vi "lights work.vi"() -> ()   [LabVIEW 2016]
doc: "ADXL362 SPI Accelerometer\n\nThis example shows how to use the Analog Devices ADXL362 Accelerometer sensor connected to SPI.\n\nThis example expects a USB cable connected from your development PC to the Type B USB Jack (next to the power input) on the roboRIO."
uses:
  <vilib>/Rock Robotics/SystemInterfaces/spilib/spi_bus.ctl
  <vilib>/Rock Robotics/WPI/SPI/WPI_SPIMode.ctl
panel:
  out "Previous":i32[](array[numeric])
  out "ONOFF":bool
  in  "Blink Rate":u32
  in  "Aiming":u32(colorbox)
  in  "Loader":bool
  in  "Intake":bool
  in  "Shooter":bool
  in  "Blinky End":u8
  in  "Chaser (Gap)":u8
  in  "Display Style":u8(knob) scale=0.0..6.0
  out "Aiming":bool
  out "Loader":bool
  out "Intake":bool
  out "Shooter":bool
  in  "Global Max\nBrightness":u8(slide) max=31 scale=0.0..31.0
  in  "Brightness B":u8
  in  "Brighness R":u8
  in  "Brigtness G":u8
  in  "Blue":bool
  in  "Red":bool
  in  "Green":bool
  in  "Number of Lights":u8
  in  "Number ON":u8
  in  "Chip Select Active High (F)":bool
  in  "Mode (3)":T1=enum."Mode 3 (Clk Idle High,Sample on Trailing)"
  in  "Clock Rate (Hz)":dbl=500000.0
  in  "error in":errorcluster
  in  "SPI Bus":T2=enum."SPI On-Board, CS1"
  out "error out":errorcluster
  in  "stop":bool
  # "Set these inputs before running."
  # "Number of Lights"
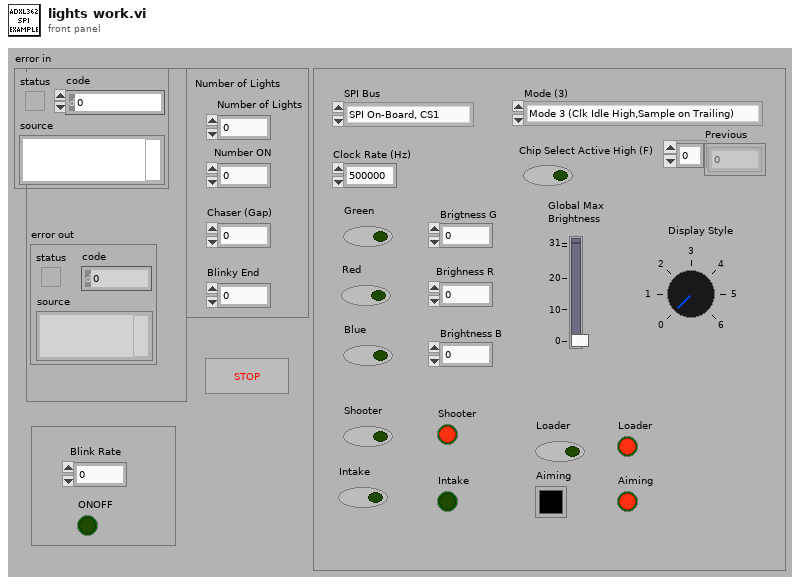
[diagram p1: front panel]
types:
  T1 = typedef "WPI_SPIMode.ctl" = enum16{"Mode 0 (Clk Idle Low,Sample on Leading)", "Mode 1 (Clk Idle Low,Sample on Trailing)", "Mode 2 (Clk Idle High,Sample on Leading)", "Mode 3 (Clk Idle High,Sample on Trailing)"}
  T2 = typedef "spi_bus.ctl" = enum16{"SPI On-Board, CS0", "SPI On-Board, CS1", "SPI On-Board, CS2", "SPI On-Board, CS3", "SPI MXP", "Invalid"}
  T3 = typedef "WPI_SPIDevRef.ctl" = cluster{"DevStatus":errorcluster, "Handle":i32, "SPI Bus":T2}
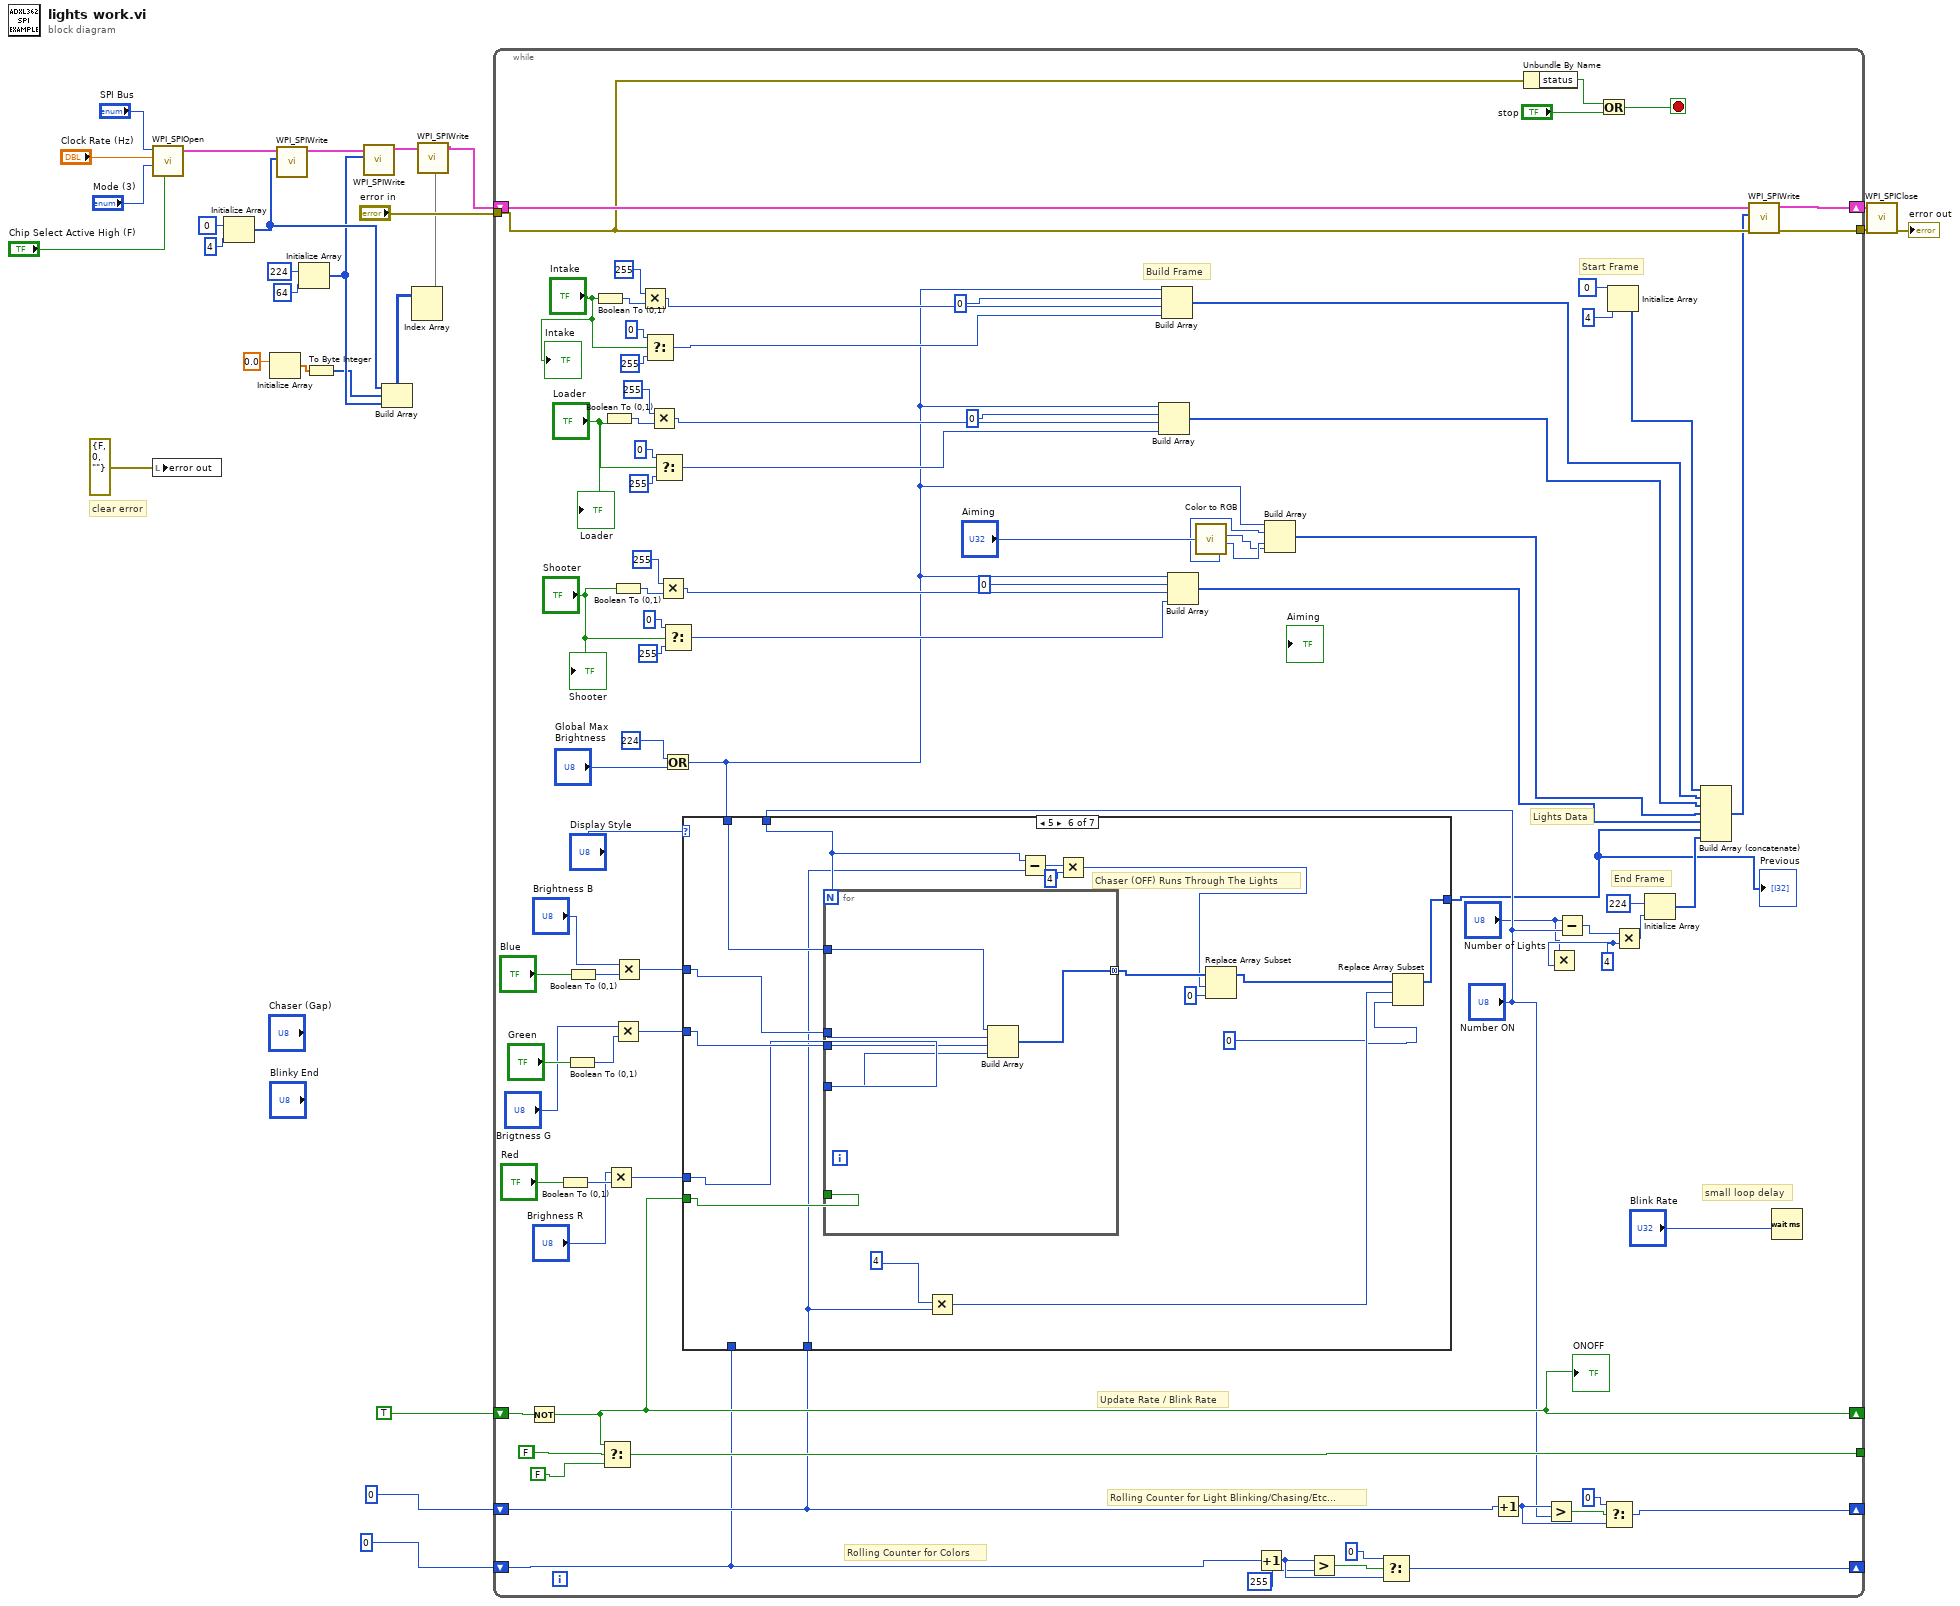
[diagram p0: block diagram]
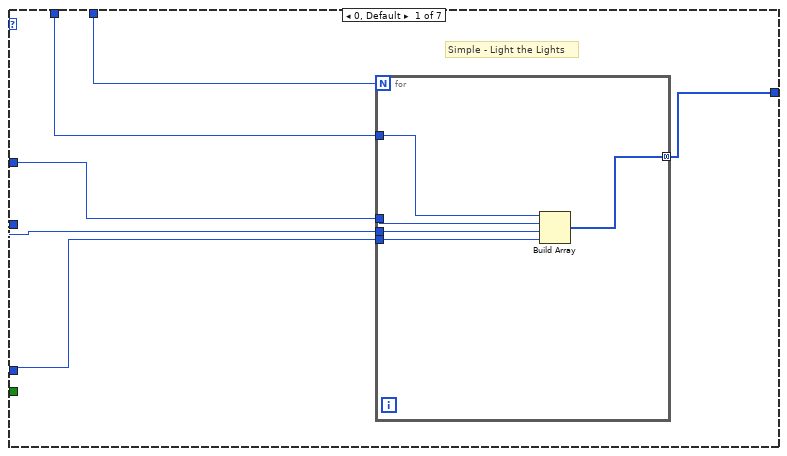
[diagram p2: hidden frame]
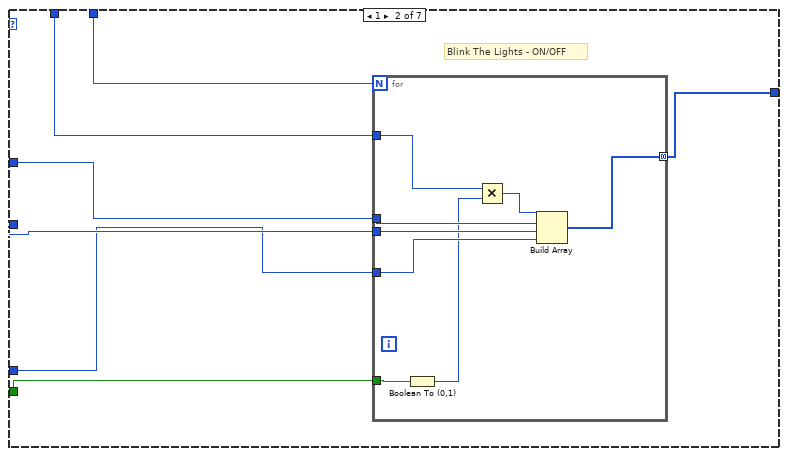
[diagram p3: hidden frame]
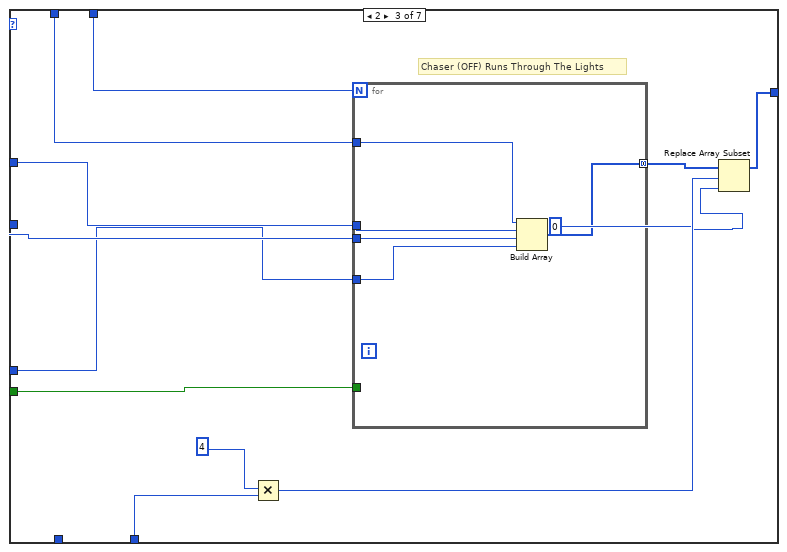
[diagram p4: hidden frame]
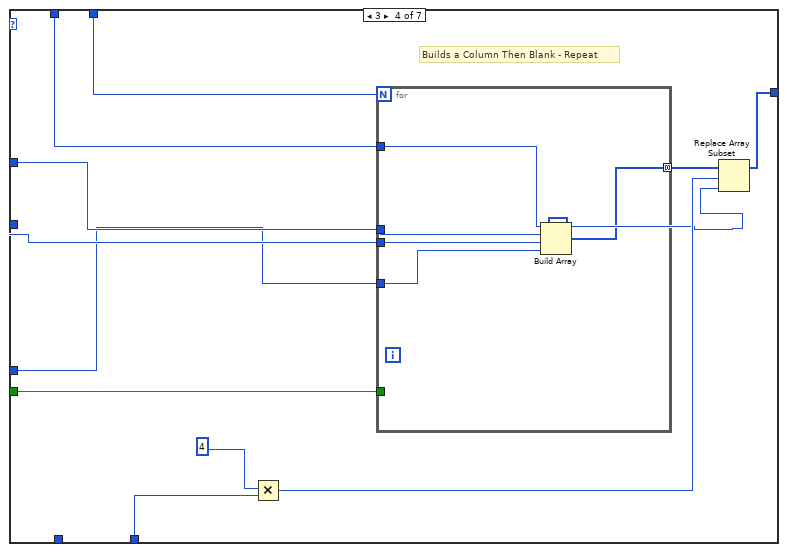
[diagram p5: hidden frame]
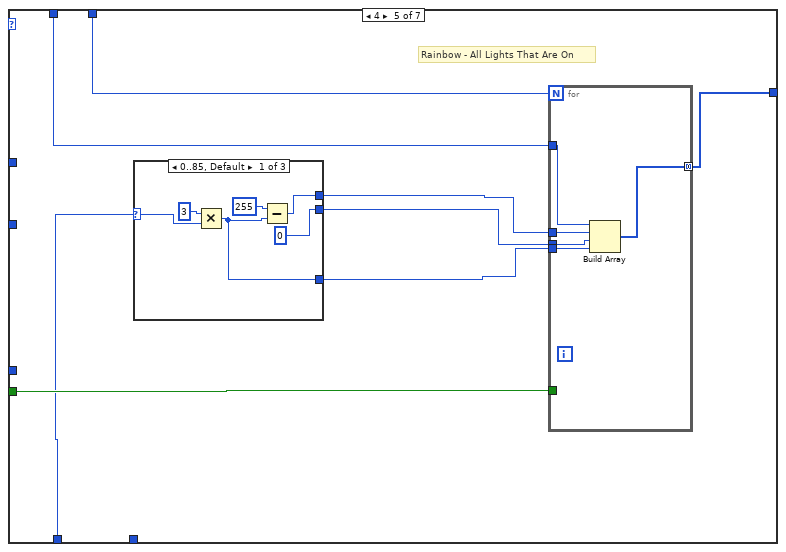
[diagram p6: hidden frame]
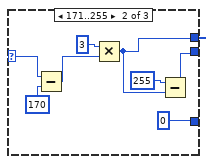
[diagram p7: hidden frame]
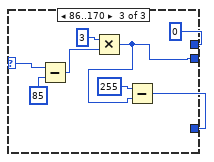
[diagram p8: hidden frame]
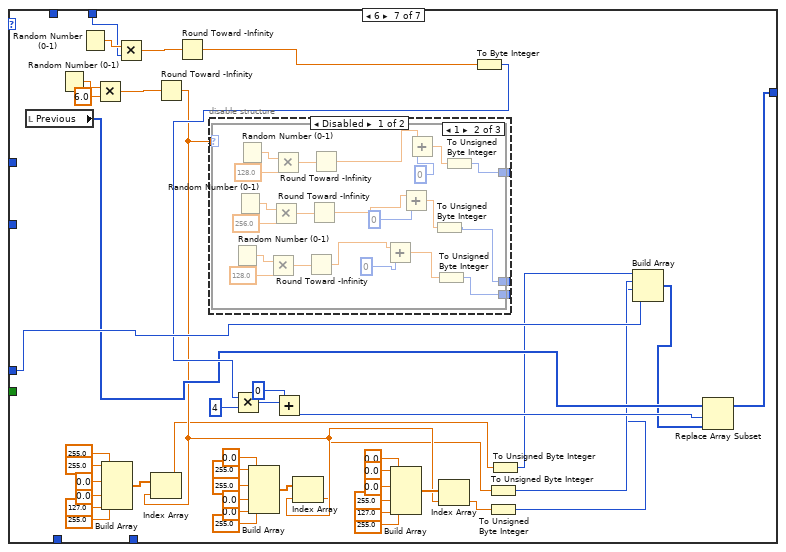
[diagram p9: hidden frame]
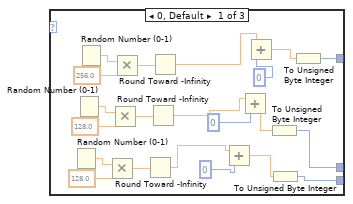
[diagram p10: hidden frame]
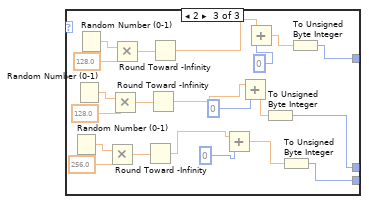
[diagram p11: hidden frame]
diagram:
  # "clear error"
  n1 = call <vilib>:"WPI_SPIOpen.vi"("Chip Select Active High (F)"="Chip Select Active High (F)", "Mode (3)"="Mode (3)", "Clock Rate (Hz)"="Clock Rate (Hz)", "SPI Bus"="SPI Bus") -> ("SPIDevRef"=w17:T3)  [unwired: 6 in, 1 out]
  n2 = local write "error out"(errorcluster {"status"=FALSE, "code"=0, "source"=""} ("error out")) -> ()
  n3 = Initialize Array(u8 0 ("Data To Send"), u8 4 ("dimension size")) -> (w9:u8[])
  n4 = Initialize Array(0.0 ("element")) -> (w4:dbl[])  [unwired: 1 in]
  n5 = call <vilib>:"WPI_SPIWrite.vi"("Data To Send"=w9, "SPIDevRef"=w17) -> ("SPIDevRef"=w13:T3)  [unwired: 7 in, 2 out]
  n6 = Initialize Array(u8 224 ("Data To Send"), u8 64 ("dimension size")) -> (w8:u8[])
  n7 = To Byte Integer(number=w4) -> (8bit integer=w3:i8[])
  n8 = call <vilib>:"WPI_SPIWrite.vi"("Data To Send"=w8, "SPIDevRef"=w13) -> ("SPIDevRef"=w6:T3)  [unwired: 7 in, 2 out]
  n9 = Build Array(w9, w3, w8) -> (w2:u8[][])
  n10 = Index Array(array=w2) -> (element=w1:u8[])  [unwired: 2 in]
  n11 = call <vilib>:"WPI_SPIWrite.vi"("Data To Send"=w1, "SPIDevRef"=w6) -> ("SPIDevRef"=w7:T3)  [unwired: 7 in, 2 out]
  n12 = while {
    shift-right: [w107] -> w24
    shift-left: w7 -> [w101]
    tunnel: "error in" -> [w98]
    tunnel: [w106] -> w14
    tunnel: [w49] -> _
    shift-right: [w47] -> _
    shift-left: TRUE -> [w48]
    shift-right: [w43] -> _
    shift-left: 0 -> [w41]
    shift-right: [w37] -> _
    shift-left: 0 -> [w35]
    stop <- w97 stop-if-true
    (unwired) TRUE
    w31 = u8 4 ("dimension size")
    # "Update Rate / Blink Rate"
    # "Rolling Counter for Light Blinking/Chasing/Etc..."
    # "Rolling Counter for Colors"
    # "Build Frame"
    # "Lights Data"
    # "End Frame"
    # "Start Frame"
    # "small loop delay"
    n13 = Not(x=w48) -> (.not. x?=w47:bool)
    "ONOFF" <- w47
    n14 = Boolean To (0,1)(Boolean="Red") -> (0, 1=w56:i16)
    n15 = Boolean To (0,1)(Boolean="Green") -> (0, 1=w57:i16)
    n16 = Boolean To (0,1)(Boolean="Blue") -> (0, 1=w58:i16)
    n17 = Boolean To (0,1)(Boolean="Intake") -> (0, 1=w94:i16)
    n18 = Select(t=w47, s=FALSE, f=FALSE) -> (s? t:f=w49:bool)
    n19 = Boolean To (0,1)(Boolean="Loader") -> (0, 1=w87:i16)
    n20 = Multiply(x="Brighness R", y=w56) -> (x*y=w54:i16)
    n21 = Boolean To (0,1)(Boolean="Shooter") -> (0, 1=w82:i16)
    n22 = Multiply(x="Brigtness G", y=w57) -> (x*y=w55:i16)
    n23 = Multiply(x="Brightness B", y=w58) -> (x*y=w53:i16)
    n24 = Multiply(x=u8 255, y=w94) -> (x*y=w76:i16)
    n25 = Select(t=u8 0, s="Intake", f=u8 255) -> (s? t:f=w77:u8)
    n26 = Multiply(x=u8 255, y=w87) -> (x*y=w74:i16)
    n27 = Select(t=u8 0, s="Loader", f=u8 255) -> (s? t:f=w73:u8)
    n28 = Multiply(x=u8 255, y=w82) -> (x*y=w71:i16)
    n29 = Select(t=u8 0, s="Shooter", f=u8 255) -> (s? t:f=w70:u8)
    n30 = Or(x=u8 224, y="Global Max\nBrightness") -> (x .or. y?=w62:u8)
    n31 = case shown="5" "Display Style" {
      tunnel: [w112 w123 w138 w155 w172 w215 w260] -> w29
      tunnel: w62 -> [w117 w129 w149 w166 w179 w216 _]
      tunnel: "Number ON" -> [w116 w128 w144 w161 w177 w212 w269]
      tunnel: w55 -> [w114 w126 w147 w164 _ w218 _]
      tunnel: w54 -> [w113 w125 w146 w163 _ w217 w265]
      tunnel: w53 -> [w115 w127 w148 w165 _ w219 _]
      tunnel: w47 -> [_ w124 w145 w162 w178 w220 _]
      tunnel: w41 -> [_ _ w143 w160 _ w211 _]
      tunnel: w35 -> [_ _ _ _ w176 _ _]
      frame 0, Default {
        # "Simple - Light the Lights"
        n32 = for {
          N: w116 -> [_]
          tunnel: [w122] -> w112 mode=concatenating
          tunnel: w117 -> [w121]
          tunnel: w115 -> [w120]
          tunnel: w114 -> [w119]
          tunnel: w113 -> [w118]
          n33 = Build Array(w121, w120, w119, w118) -> (w122:i16[])
        }
      }
      frame 1 {
        # "Blink The Lights - ON/OFF"
        n34 = for {
          N: w128 -> [_]
          tunnel: [w137] -> w123 mode=concatenating
          tunnel: w129 -> [w132]
          tunnel: w127 -> [w136]
          tunnel: w126 -> [w135]
          tunnel: w125 -> [w134]
          tunnel: w124 -> [w133]
          n35 = Boolean To (0,1)(Boolean=w133) -> (0, 1=w131:i16)
          n36 = Multiply(x=w132, y=w131) -> (x*y=w130:i16)
          n37 = Build Array(w130, w136, w135, w134) -> (w137:i16[])
        }
      }
      frame 2 {
        # "Chaser (OFF) Runs Through The Lights"
        n38 = Multiply(x=4, y=w143) -> (x*y=w140:i32)
        n39 = for {
          N: w144 -> [_]
          tunnel: [w154] -> w141 mode=concatenating
          tunnel: w149 -> [w150]
          tunnel: w148 -> [w153]
          tunnel: w147 -> [w152]
          tunnel: w146 -> [w151]
          tunnel: w145 -> [_]
          n40 = Build Array(w150, w153, w152, w151) -> (w154:i16[])
        }
        n41 = Replace Array Subset(array=w141, new element=u8 0, index=w140) -> (w138:i16[])
      }
      frame 3 {
        # "Builds a Column Then Blank - Repeat"
        n42 = Multiply(x=4, y=w160) -> (x*y=w157:i32)
        n43 = for {
          N: w161 -> [_]
          tunnel: [w171] -> w158 mode=concatenating
          tunnel: w166 -> [w167]
          tunnel: w165 -> [w170]
          tunnel: w164 -> [w169]
          tunnel: w163 -> [w168]
          tunnel: w162 -> [_]
          n44 = Build Array(w167, w170, w169, w168) -> (w171:i16[])
        }
        n45 = Replace Array Subset(array=w158, new element=u8 224, index=w157) -> (w155:i16[])
      }
      frame 4 {
        # "Rainbow - All Lights That Are On"
        n46 = case shown="0..85, Default" w176 {
          selector: w176 -> [w181 w190 w199]
          tunnel: [w183 w186 0] -> w175
          tunnel: [0 w188 w194] -> w174
          tunnel: [w180 0 w195] -> w173
          frame 0..85, Default {
            n47 = Multiply(x=3, y=w181) -> (x*y=w180:i32)
            n48 = Subtract(x=255, y=w180) -> (x-y=w183:i32)
          }
          frame 171..255 {
            n49 = Subtract(x=w190, y=170) -> (x-y=w187:i32)
            n50 = Multiply(x=3, y=w187) -> (x*y=w186:i32)
            n51 = Subtract(x=255, y=w186) -> (x-y=w188:i32)
          }
          frame 86..170 {
            n52 = Subtract(x=w199, y=85) -> (x-y=w196:i32)
            n53 = Multiply(x=3, y=w196) -> (x*y=w194:i32)
            n54 = Subtract(x=255, y=w194) -> (x-y=w195:i32)
          }
        }
        n55 = for {
          N: w177 -> [_]
          tunnel: [w206] -> w172 mode=concatenating
          tunnel: w179 -> [w205]
          tunnel: w178 -> [_]
          tunnel: w175 -> [w204]
          tunnel: w174 -> [w203]
          tunnel: w173 -> [w202]
          n56 = Build Array(w205, w204, w203, w202) -> (w206:i32[])
        }
      }
      frame 5 {
        # "Chaser (OFF) Runs Through The Lights"
        n57 = for {
          N: w212 -> [_]
          tunnel: [w228] -> w214 mode=concatenating
          tunnel: w216 -> [w224]
          tunnel: w219 -> [w227]
          tunnel: w218 -> [w226]
          tunnel: w217 -> [w225]
          tunnel: w220 -> [_]
          n58 = Build Array(w224, w227, w226, w225) -> (w228:i16[])
        }
        n59 = Multiply(x=4, y=w211) -> (x*y=w222:i32)
        n60 = Subtract(x=w212, y=w211) -> (x-y=w210:i32)
        n61 = Multiply(x=w210, y=4) -> (x*y=w208:i32)
        n62 = Replace Array Subset(array=w214, new element=i16 0 ("new element/subarray"), index=w208) -> (w213:i16[])
        n63 = Replace Array Subset(array=w213, new element=u8 0, index=w222) -> (w215:i16[])
      }
      frame 6 {
        n64 = local read "Previous"() -> (w259:i32[])
        n65 = Random Number (0-1)() -> (number: 0 to 1=w262:dbl)
        n66 = Random Number (0-1)() -> (number: 0 to 1=w271:dbl)
        n67 = Multiply(x=w262, y=6.0) -> (x*y=w263:dbl)
        n68 = Build Array(255.0 ("element"), 255.0 ("element"), 0.0 ("element"), 0.0 ("element"), 127.0 ("element"), 255.0 ("element")) -> (w238:dbl[])
        n69 = Multiply(x=w271, y=w269) -> (x*y=w272:dbl)
        n70 = Round Toward -Infinity(1:w263) -> (0:w235:dbl)
        n71 = Index Array(array=w238, index=w235) -> (element=w234:dbl)
        n72 = Round Toward -Infinity(1:w272) -> (0:w270:dbl)
        n73 = disable-structure shown="Disabled" {
          disable-tunnel: w235 -> [w276 _]
          disable-tunnel: [w275 _] -> _
          disable-tunnel: [w274 _] -> _
          disable-tunnel: [w273 _] -> _
          frame Disabled {
            n74 = case shown="1" w276 {
              tunnel: [w282 w302 w323] -> w275
              tunnel: [w279 w300 w321] -> w274
              tunnel: [w278 w298 w319] -> w273
              frame 0, Default {
                n75 = Random Number (0-1)() -> (number: 0 to 1=w285:dbl)
                n76 = Random Number (0-1)() -> (number: 0 to 1=w288:dbl)
                n77 = Random Number (0-1)() -> (number: 0 to 1=w292:dbl)
                n78 = Multiply(x=w285, y=128.0) -> (x*y=w286:dbl)
                n79 = Multiply(x=w288, y=128.0) -> (x*y=w289:dbl)
                n80 = Multiply(x=w292, y=256.0) -> (x*y=w291:dbl)
                n81 = Round Toward -Infinity(1:w286) -> (0:w294:dbl)
                n82 = Round Toward -Infinity(1:w289) -> (0:w293:dbl)
                n83 = Round Toward -Infinity(1:w291) -> (0:w283:dbl)
                n84 = Add(x=w294, y=0) -> (x+y=w277:dbl)
                n85 = Add(x=w293, y=0) -> (x+y=w280:dbl)
                n86 = Add(x=w283, y=0) -> (x+y=w281:dbl)
                n87 = To Unsigned Byte Integer(number=w280) -> (unsigned 8bit integer=w279:u8)
                n88 = To Unsigned Byte Integer(number=w277) -> (unsigned 8bit integer=w278:u8)
                n89 = To Unsigned Byte Integer(number=w281) -> (unsigned 8bit integer=w282:u8)
              }
              frame 1 {
                n90 = Random Number (0-1)() -> (number: 0 to 1=w306:dbl)
                n91 = Random Number (0-1)() -> (number: 0 to 1=w309:dbl)
                n92 = Random Number (0-1)() -> (number: 0 to 1=w313:dbl)
                n93 = Multiply(x=w306, y=128.0) -> (x*y=w307:dbl)
                n94 = Multiply(x=w309, y=256.0) -> (x*y=w310:dbl)
                n95 = Multiply(x=w313, y=128.0) -> (x*y=w312:dbl)
                n96 = Round Toward -Infinity(1:w307) -> (0:w315:dbl)
                n97 = Round Toward -Infinity(1:w310) -> (0:w314:dbl)
                n98 = Round Toward -Infinity(1:w312) -> (0:w304:dbl)
                n99 = Add(x=w315, y=0) -> (x+y=w299:dbl)
                n100 = Add(x=w314, y=0) -> (x+y=w301:dbl)
                n101 = Add(x=w304, y=0) -> (x+y=w303:dbl)
                n102 = To Unsigned Byte Integer(number=w301) -> (unsigned 8bit integer=w300:u8)
                n103 = To Unsigned Byte Integer(number=w299) -> (unsigned 8bit integer=w298:u8)
                n104 = To Unsigned Byte Integer(number=w303) -> (unsigned 8bit integer=w302:u8)
              }
              frame 2 {
                n105 = Random Number (0-1)() -> (number: 0 to 1=w327:dbl)
                n106 = Random Number (0-1)() -> (number: 0 to 1=w330:dbl)
                n107 = Random Number (0-1)() -> (number: 0 to 1=w334:dbl)
                n108 = Multiply(x=w327, y=256.0) -> (x*y=w328:dbl)
                n109 = Multiply(x=w330, y=128.0) -> (x*y=w331:dbl)
                n110 = Multiply(x=w334, y=128.0) -> (x*y=w333:dbl)
                n111 = Round Toward -Infinity(1:w328) -> (0:w336:dbl)
                n112 = Round Toward -Infinity(1:w331) -> (0:w335:dbl)
                n113 = Round Toward -Infinity(1:w333) -> (0:w325:dbl)
                n114 = Add(x=w336, y=0) -> (x+y=w320:dbl)
                n115 = Add(x=w335, y=0) -> (x+y=w322:dbl)
                n116 = Add(x=w325, y=0) -> (x+y=w324:dbl)
                n117 = To Unsigned Byte Integer(number=w322) -> (unsigned 8bit integer=w321:u8)
                n118 = To Unsigned Byte Integer(number=w320) -> (unsigned 8bit integer=w319:u8)
                n119 = To Unsigned Byte Integer(number=w324) -> (unsigned 8bit integer=w323:u8)
              }
            }
          }
          frame Enabled {
          }
        }
        n120 = Build Array(255.0 ("element"), 0.0 ("element"), 255.0 ("element"), 0.0 ("element"), 0.0 ("element"), 255.0 ("element")) -> (w237:dbl[])
        n121 = Index Array(array=w237, index=w235) -> (element=w233:dbl)
        n122 = Build Array(0.0 ("element"), 0.0 ("element"), 0.0 ("element"), 255.0 ("element"), 127.0 ("element"), 255.0 ("element")) -> (w236:dbl[])
        n123 = Index Array(array=w236, index=w235) -> (element=w232:dbl)
        n124 = To Byte Integer(number=w270) -> (8bit integer=w264:i8)
        n125 = Multiply(x=w264, y=4) -> (x*y=w267:i32)
        n126 = Add(x=w267, y=0) -> (x+y=w258:i32)
        n127 = To Unsigned Byte Integer(number=w233) -> (unsigned 8bit integer=w230:u8)
        n128 = To Unsigned Byte Integer(number=w232) -> (unsigned 8bit integer=w229:u8)
        n129 = To Unsigned Byte Integer(number=w234) -> (unsigned 8bit integer=w231:u8)
        n130 = Build Array(w231, w230, w229, w265) -> (w257:i16[])
        n131 = Replace Array Subset(array=w259, new element=w257, index=w258) -> (w260:i32[])
      }
    }
    "Previous" <- w29
    n132 = Build Array(w62, u8 0, w74, w73) -> (w84:i16[])
    n133 = Build Array(w62, u8 0, w76, w77) -> (w90:i16[])
    n134 = Build Array(w62, u8 0, w71, w70) -> (w79:i16[])
    n135 = call <vilib>:"Color to RGB.vi"("Color"="Aiming") -> ("R"=w67:u8, "G"=w68:u8, "B"=w69:u8)  [unwired: 1 out]
    n136 = Increment(x=w35) -> (x+1=w38:u8)
    n137 = Build Array(w62, w69, w68, w67) -> (w89:u8[])
    n138 = Greater?(x=w38, y=255) -> (0:w39:bool)
    n139 = Select(t=0, s=w39, f=w38) -> (s? t:f=w37:i32)
    n140 = Increment(x=w41) -> (x+1=w44:u8)
    n141 = Unbundle By Name(w98) -> ("status"=w99:bool)
    n142 = Greater?(x=w44, y="Number ON") -> (0:w45:bool)
    n143 = Multiply(x="Number of Lights", y=w31) -> ()  [unwired: 1 out]
    n144 = Subtract(x="Number of Lights", y="Number ON") -> (x-y=w102:u8)
    n145 = Or(x=w99, y="stop") -> (x .or. y?=w97:bool)
    n146 = Select(t=0, s=w45, f=w44) -> (s? t:f=w43:i32)
    n147 = Initialize Array(u8 0 ("Data To Send"), u8 4 ("dimension size")) -> (w91:u8[])
    n148 = Multiply(x=w102, y=w31) -> (x*y=w103:u8)
    n149 = Initialize Array(u8 224 ("Data To Send"), w103) -> (w100:u8[])
    n150 = Build Array (concatenate)(w91, w90, w84, w89, w79, w29, w100) -> (w28:i32[])
    n151 = call <vilib>:"WPI_SPIWrite.vi"("error in (no error)"=w98, "Data To Send"=w28, "SPIDevRef"=w101) -> ("error out"=w106:errorcluster, "SPIDevRef"=w107:T3)  [unwired: 6 in, 1 out]
    n152 = Wait (ms)(milliseconds to wait="Blink Rate") -> ()  [unwired: 1 out]
    "Shooter" <- "Shooter"
    "Loader" <- "Loader"
    "Intake" <- "Intake"
  }
  n153 = call <vilib>:"WPI_SPIClose.vi"("error in (no error)"=w14, "SPIDevRef"=w24) -> ("error out"=→"error out":errorcluster)  [unwired: 9 in]
